vi "Joystick Conditioning.vi"(8 "axis 4 (a) in":dbl, 9 "axis 3 (z) in":dbl, 10 "axis 2 (y) in":dbl, 11 "axis 1 (x) in":dbl) -> (0 "axis 4 (a) out":dbl, 1 "axis 3 (z) out":dbl, 2 "axis 2 (y) out":dbl, 3 "axis 1 (x) out":dbl)   [LabVIEW 2015]
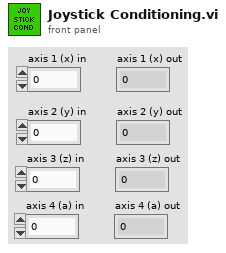
[diagram p1: front panel]
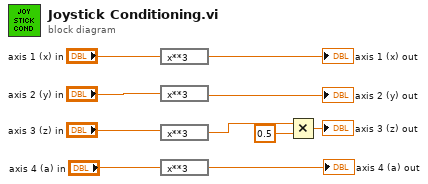
[diagram p0: block diagram]
diagram:
  n1 = expression code="x**3"("axis 1 (x) in") -> (→"axis 1 (x) out":dbl)
  n2 = expression code="x**3"("axis 2 (y) in") -> (→"axis 2 (y) out":dbl)
  n3 = expression code="x**3"("axis 3 (z) in") -> (w2:dbl)
  n4 = expression code="x**3"("axis 4 (a) in") -> (→"axis 4 (a) out":dbl)
  n5 = Multiply(x=w2, y=0.5) -> (x*y=→"axis 3 (z) out":dbl)
